vi "BinaryData.vi"() -> ()   [LabVIEW 2016]
uses:
  <vilib>/Platform/TimedLoop/XDataNode/timing_clust.ctl
  <vilib>/Platform/TimedLoop/XDataNode/nitl_modes.ctl
  <vilib>/Platform/TimedLoop/XDataNode/wakeup.ctl
  <vilib>/Utility/file.llb/Write Delimited Spreadsheet (DBL).vi
  <vilib>/Platform/TimedLoop/XDataNode/XDataNode.xnode
  <vilib>/Platform/TimedLoop/XDataNode/XDNodeRunTimeDep.lvlib
panel:
  in  "Read .bin":path=path "C:/Users/YZ/Desktop/.bin"
  in  "Write .csv":path=path "C:/Users/YZ/Desktop/.csv"
  out "Read Monitor":dbl[][](array[numeric])
  out "data":cluster{dbl[]}[](array[cluster])
  out "Write Monitor":dbl[](array[numeric])
  in  "Enum":enum16{"Read", "Write"}(ring)
  in  "stop":bool
  # "C:\\Users\\YZ\\Desktop"
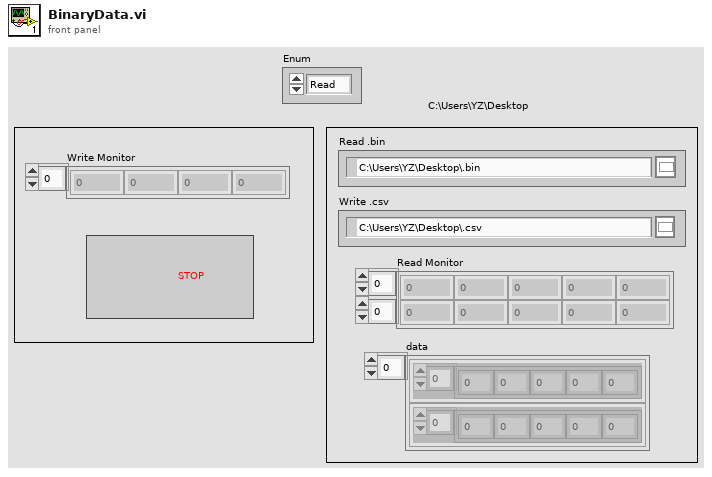
[diagram p1: front panel]
types:
  T1 = enum16{"open", "replace", "create", "open or create", "replace or create", "replace or create with confirmation"}
  T2 = typedef "XDNodeRunTimeDep.lvlib/timing_clust.ctl" = cluster{"Expected End [f-1]":u64, "Actual End [f-1]":u64, "Finished Late? [f-1]":bool, "Expected End [i-1]":u64, "Actual End [i-1]":u64, "Finished Late? [i-1]":bool, "Expected Start [i]":u64, "Actual Start [i]":u64, "Expected Start [f]":u64, "Actual Start [f]":u64, "Source Name":string, "Structure Name":string, "Period":i64, "Deadline":i64, "Offset":i64, "Start":i64, "Priority":i32, "Timeout":i32, "Mode":T3, "Wakeup Reason":T4, "Error":errorcluster, "Source Type":string, "Secondary Source Type":string, "Global End Time":u64, "Global Start Time":u64, "Frame Duration":u64, "Iteration Duration":u64, "Assigned CPU":i32, "I/O Scan Engine Mode":u32}
  T3 = typedef "XDNodeRunTimeDep.lvlib/nitl_modes.ctl" = enum32{"No Change", "Process missed periods, maintain original phase", "Discard missed periods, maintain original phase", "Process missed periods, ignore original phase", "Discard missed periods, ignore original phase"}
  T4 = typedef "XDNodeRunTimeDep.lvlib/wakeup.ctl" = enum32{"Normal", "Aborted", "Asynchronous wakeup", "Timing source error", "Timed loop error", "Timeout"}
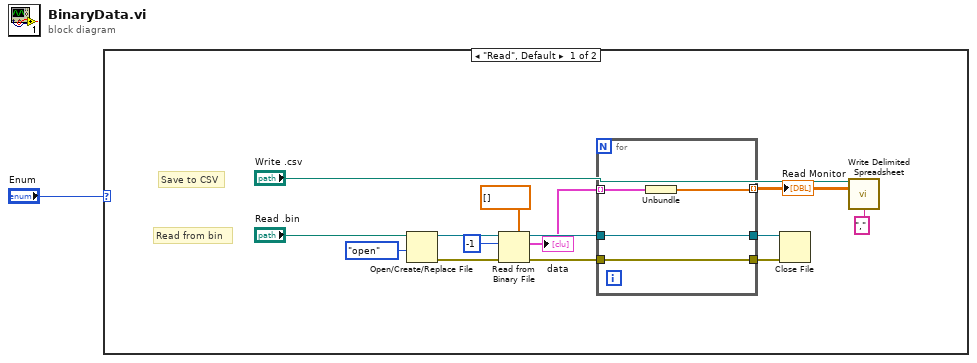
[diagram p0: block diagram]
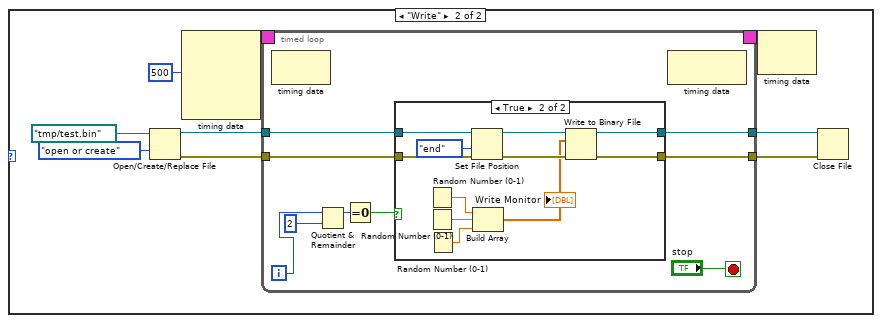
[diagram p2: hidden frame]
diagram:
  n1 = case shown="\"Read\", Default" "Enum" {
    frame "Read", Default {
      # "Read from bin"
      # "Save to CSV"
      n2 = Open/Create/Replace File(file path (use dialog)="Read .bin", operation (0:open)=T1."open") -> (refnum out=w7:refnum<file>, error out=w6:errorcluster)  [unwired: 4 in, 1 out]
      n3 = Read from Binary File(5:dbl[] [], 8:w6, 10:-1 ("count (1)"), 11:w7) -> (0:w9:errorcluster, 2:w4:cluster{dbl[]}[], 3:w11:refnum<file>)  [unwired: 2 in, 1 out]
      "data" <- w4
      n4 = for {
        tunnel: w4 -> [w17] mode=indexing
        tunnel: w11 -> [w19]
        tunnel: [w19] -> w10
        tunnel: w9 -> [w18]
        tunnel: [w18] -> w8
        tunnel: [w16] -> w2 mode=indexing
        n5 = Unbundle(w17) -> (w16:dbl[])
      }
      "Read Monitor" <- w2
      n6 = Close File(refnum=w10, error in=w8) -> ()  [unwired: 2 out]
      n7 = call-poly <vilib>:"Write Delimited Spreadsheet.vi"("file path (dialog if empty)"="Write .csv", "2D data"=w2, "delimiter (\\t)"="," ("delimiter (\\t)")) -> ()  [unwired: 11 in, 2 out]
    }
    frame "Write" {
      n8 = Open/Create/Replace File(file path (use dialog)=path "/tmp/test.bin", operation (0:open)=T1."open or create") -> (refnum out=w23:refnum<file>, error out=w24:errorcluster)  [unwired: 4 in, 1 out]
      n9 = node-c288(i64 500 ("Period")) -> (w22:T2)  [unwired: 3 in]
      n10 = timed-loop {
        tunnel: w23 -> [w34]
        tunnel: [w37] -> w25
        tunnel: w24 -> [w33]
        tunnel: [w36] -> w26
        timing: w22 -> [_]
        timing-out: [_] -> w21
        i -> [w30]
        stop <- "stop" stop-if-true
        n11 = node-c288() -> ()  [unwired: 1 in, 1 out]
        n12 = Quotient & Remainder(x=w30, y=2) -> (x-y*floor(x/y)=w31:i32)  [unwired: 1 out]
        n13 = Equal To 0?(x=w31) -> (x = 0?=w29:bool)
        n14 = case shown="True" w29 {
          tunnel: [w39 w50] -> w37
          tunnel: [w38 w49] -> w36
          tunnel: w34 -> [w39 w45]
          tunnel: w33 -> [w38 w43]
          frame False {
          }
          frame True {
            n15 = Random Number (0-1)() -> (number: 0 to 1=w48:dbl)
            n16 = Random Number (0-1)() -> (number: 0 to 1=w47:dbl)
            n17 = Random Number (0-1)() -> (number: 0 to 1=w46:dbl)
            n18 = Set File Position(refnum=w45, from (0:start)=enum16{"start", "end", "current"}."end", error in=w43) -> (refnum out=w44:refnum<file>, error out=w42:errorcluster)  [unwired: 1 in]
            n19 = Build Array(w48, w47, w46) -> (w40:dbl[])
            "Write Monitor" <- w40
            n20 = Write to Binary File(file (use dialog)=w44, data=w40, error in=w42) -> (refnum out=w50:refnum<file>, error out=w49:errorcluster)  [unwired: 3 in, 1 out]
          }
        }
        n21 = node-c288() -> ()  [unwired: 1 in, 1 out]
      }
      n22 = node-c288(w21) -> ()  [unwired: 1 out]
      n23 = Close File(refnum=w25, error in=w26) -> ()  [unwired: 2 out]
    }
  }
